vi "Configure IMD proto settings.vi"(11 "measurement configuration":T1={"Full scale range"=2.825, "Channel name"="", "Analog source resource name"="", "IMD standard"=enum."SMPTE (60 Hz, 7000 Hz, 4:1)", "Low frequency"=0.0, "High frequency"=0.0, "Amplitude ratio"=0.0, "Amplitude"=0.0, "Protocol capture resource name"="", "Data line"=0, "Channel"=0, "Sample rate"=44100.0, "Measurement duration"=0.1, "Frame sync edge for Channel 0"=enum."Falling", "Channel count per frame"=2, "Channel length"=32, "Bit depth"=24, "Channel 0 offset"=1, "Endianness"=enum."MSB First", "Data Justification"=enum."Left Justified", "Frame length"=64, "Frame sync pulse width"=32, "Bit clock edge  sync"=enum."Falling"}) -> (3 "Protocol settings":T2={"Protocol capture resource name"="", "Data line"=0, "Channel"="", "Clock rate"=12288000, "Number of words"=19200, "Sensitivity"=0.34762, "Frame sync edge for channel 0"=enum."Falling", "Channel count per frame"=2, "Channel length"=32, "Bit depth"=24, "Channel 0 offset"=1, "Endianness"=enum."MSB First", "Data justification"=enum."Left Justified", "Frame length"=64, "Frame sync pulse width"=32, "Bit clock edge sync"=enum."Falling"})   [LabVIEW 2021, in "IMD_Audio ADC.lvlib"]
uses:
  IMD_Audio ADC.lvlib
  shared/controls/Protocol Settings Dual Channel.ctl
  Measurement Configuration.ctl
  shared/controls/Audio ADC Controls.lvlib
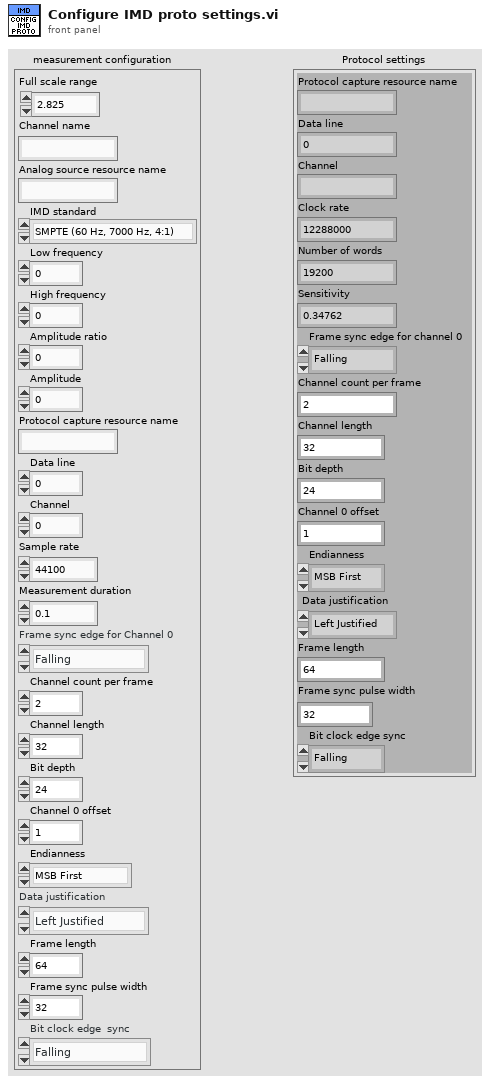
[diagram p1: front panel]
types:
  T1 = typedef "IMD_Audio ADC.lvlib/Measurement Configuration.ctl" = cluster{"Full scale range":dbl, "Channel name":string, "Analog source resource name":string, "IMD standard":enum32{"SMPTE (60 Hz, 7000 Hz, 4:1)", "DIN (250 Hz, 8000 Hz, 4:1)", "CCIF (11 kHz, 12 kHz, 1:1)", "CCIF (19 kHz, 20 kHz, 1:1)", "Custom"}, "Low frequency":dbl, "High frequency":dbl, "Amplitude ratio":dbl, "Amplitude":dbl, "Protocol capture resource name":string, "Data line":u32, "Channel":u32, "Sample rate":dbl, "Measurement duration":dbl, "Frame sync edge for Channel 0":enum32{"Rising", "Falling"}, "Channel count per frame":u32, "Channel length":u32, "Bit depth":u32, "Channel 0 offset":u32, "Endianness":enum32{"MSB First", "LSB First"}, "Data Justification":enum32{"Left Justified", "Right Justified"}, "Frame length":u32, "Frame sync pulse width":u32, "Bit clock edge  sync":enum32{"Rising", "Falling"}}
  T2 = typedef "Audio ADC Controls.lvlib/Protocol Settings Dual Channel.ctl" = cluster{"Protocol capture resource name":string, "Data line":u16, "Channel":string, "Clock rate":u32, "Number of words":i32, "Sensitivity":dbl, "Frame sync edge for channel 0":enum32{"Rising", "Falling"}, "Channel count per frame":u8, "Channel length":u16, "Bit depth":u8, "Channel 0 offset":u16, "Endianness":enum32{"MSB First", "LSB First"}, "Data justification":enum32{"Left Justified", "Right Justified"}, "Frame length":u16, "Frame sync pulse width":u16, "Bit clock edge sync":enum32{"Rising", "Falling"}}
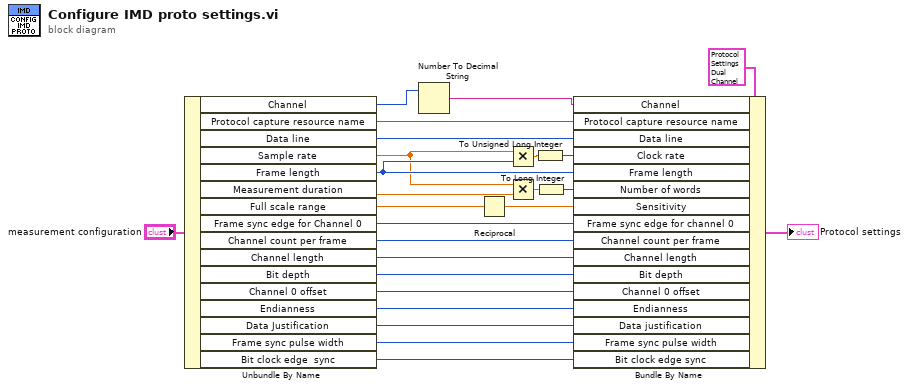
[diagram p0: block diagram]
diagram:
  n1 = Unbundle By Name("measurement configuration") -> ("Channel"=w3:u32, "Protocol capture resource name"=w24:string, "Data line"=w23:u32, "Sample rate"=w9:dbl, "Frame length"=w11:u32, "Measurement duration"=w10:dbl, "Full scale range"=w6:dbl, "Frame sync edge for Channel 0"=w14:enum32{"Rising", "Falling"}, "Channel count per frame"=w22:u32, "Channel length"=w21:u32, "Bit depth"=w20:u32, "Channel 0 offset"=w19:u32, "Endianness"=w18:enum32{"MSB First", "LSB First"}, "Data Justification"=w17:enum32{"Left Justified", "Right Justified"}, "Frame sync pulse width"=w16:u32, "Bit clock edge  sync"=w15:enum32{"Rising", "Falling"})
  n2 = Number To Decimal String(number=w3) -> (decimal integer string=w2:string)  [unwired: 1 in]
  n3 = Reciprocal(x=w6) -> (1/x=w5:dbl)
  n4 = Multiply(x=w9, y=w11) -> (x*y=w13:dbl)
  n5 = Multiply(x=w9, y=w10) -> (x*y=w8:dbl)
  n6 = To Unsigned Long Integer(number=w13) -> (unsigned 32bit integer=w12:u32)
  n7 = To Long Integer(number=w8) -> (32bit integer=w7:i32)
  n8 = Bundle By Name(cluster=T2 {"Protocol capture resource name"="", "Data line"=0, "Channel"="", "Clock rate"=12288000, "Number of words"=19200, "Sensitivity"=0.34762, "Frame sync edge for channel 0"=enum."Falling", "Channel count per frame"=2, "Channel length"=32, "Bit depth"=24, "Channel 0 offset"=1, "Endianness"=enum."MSB First", "Data justification"=enum."Left Justified", "Frame length"=64, "Frame sync pulse width"=32, "Bit clock edge sync"=enum."Falling"} ("Protocol settings"), "Channel"=w2, "Protocol capture resource name"=w24, "Data line"=w23, "Clock rate"=w12, "Frame length"=w11, "Number of words"=w7, "Sensitivity"=w5, "Frame sync edge for channel 0"=w14, "Channel count per frame"=w22, "Channel length"=w21, "Bit depth"=w20, "Channel 0 offset"=w19, "Endianness"=w18, "Data justification"=w17, "Frame sync pulse width"=w16, "Bit clock edge sync"=w15) -> (→"Protocol settings":T2)
